vi "robo_waitEnd.vi"(0 "VISA资源名称":refnum<visa-resource-name>, 1 "ax":i32, 2 "page":i32, 3 "错误输入（无错误）":errorcluster, 4 "tmo":i32=60000) -> (5 "VISA资源名称输出":refnum<visa-resource-name>, 6 "f":i32, 7 "错误输出":errorcluster)   [LabVIEW 2017]
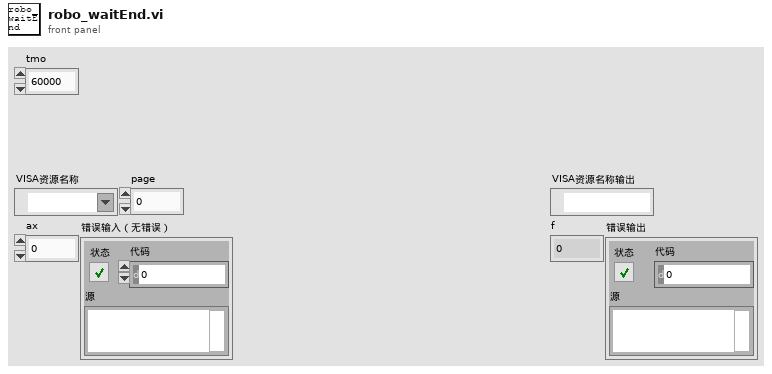
[diagram p1: front panel]
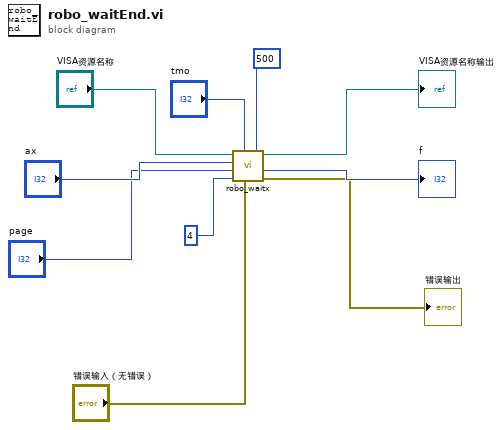
[diagram p0: block diagram]
diagram:
  n1 = call "robo_waitx.vi"("tick"=500, "错误输入（无错误）"="错误输入（无错误）", "tmo"="tmo", "dst"=4, "page"="page", "ax"="ax", "VISA资源名称"="VISA资源名称") -> ("错误输出"=→"错误输出":errorcluster, "f"=→"f":i32, "VISA资源名称输出"=→"VISA资源名称输出":refnum<visa-resource-name>)
